vi "createSheet.vi"(6 "Set as active (T)":bool=TRUE, 8 "error in (no error)":errorcluster, 10 "SheetName":string, 11 "MS-Excel in":refnum<class "MS-Excel.lvclass">) -> (0 "error out":errorcluster, 1 "Created?":bool, 2 "Created Sheet Name":string, 3 "MS-Excel out":refnum<class "MS-Excel.lvclass">)   [LabVIEW 2020, in "LabVIEW NPOI.lvlib" / "MS-Excel.lvclass"]
uses:
  MS-Excel.lvclass
  D:/Benjamin/Documents/Perso/Code/WC/LabVIEW_NPOI/lib/NPOI 2.1.1/NPOI.dll
  lib/NPOI 2.1.1/NPOI.dll
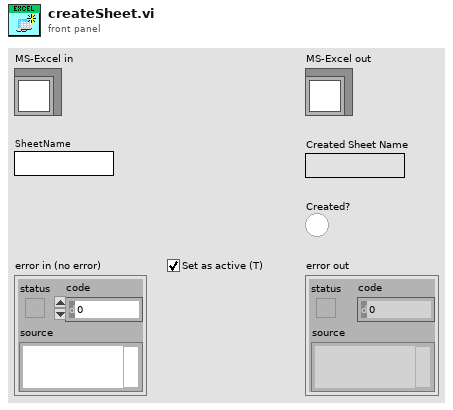
[diagram p1: front panel]
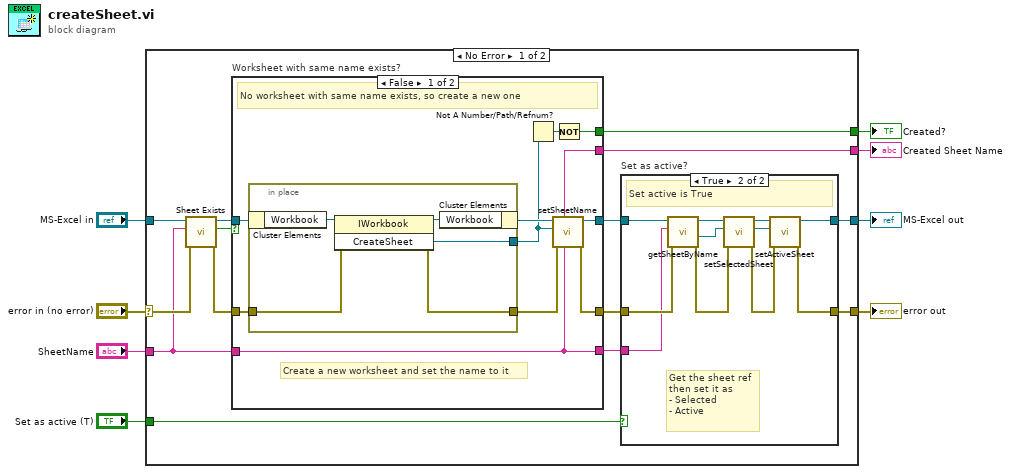
[diagram p0: block diagram]
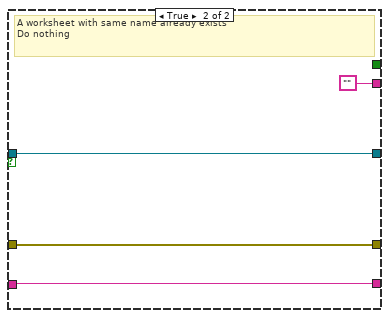
[diagram p3: hidden frame]
diagram:
  n1 = case shown="No Error" "error in (no error)" {
    selector: "error in (no error)" -> [w19 w55]
    tunnel: [w13 w55] -> w7
    tunnel: [w12 w54] -> w5
    tunnel: "MS-Excel in" -> [w22 w54]
    tunnel: "SheetName" -> [w17 _]
    tunnel: "Set as active (T)" -> [w11 _]
    tunnel: [w21 _] -> w2
    tunnel: [w9 _] -> w1
    frame No Error {
      n2 = call "Sheet Exists.vi"("error in (no error)"=w19, "Sheet Name"=w17, "MS-Excel in"=w22) -> ("error out"=w18:errorcluster, "Exists"=w16:bool, "MS-Excel out"=w20:refnum<class "MS-Excel.lvclass">)  [unwired: 6 in]
      n3 = case "Worksheet with same name exists?" shown="False" w16 {
        tunnel: [w36 w53] -> w15
        tunnel: [w37 w52] -> w14
        tunnel: [w42 _] -> w21
        tunnel: w20 -> [w39 w53]
        tunnel: w17 -> [w35 w51]
        tunnel: w18 -> [w38 w52]
        tunnel: [w35 w51] -> w10
        tunnel: [w35 "" ("SheetName")] -> w9
        frame False {
          # "Create a new worksheet and set the name to it"
          # "No worksheet with same name exists, so create a new one"
          n4 = in-place {
            in-place-border: w38 -> [w48]
            in-place-border: [w46] -> w40
            in-place-border: [w45] -> w41
            n5 = in-place-cluster #1(w39) -> ("Workbook"=w49:refnum<k24>)
            n6 = invoke class="IWorkbook" method="CreateSheet"(reference=w49, error in=w48) -> (reference out=w47:refnum<k24>, error out=w46:errorcluster, "CreateSheet"=w45:refnum<k24>)  [unwired: 1 in]
            n7 = in-place-cluster #1("Workbook"=w47) -> (w44:refnum<class "MS-Excel.lvclass">)
          }
          n8 = Not A Number/Path/Refnum?(number/path/refnum=w41) -> (NaN/Path/Refnum?=w43:bool)
          n9 = call-dynamic "setSheetName.vi"("Sheet Name"=w35, "error in (no error)"=w40, "SheetRef"=w41, "MS-Excel in"=w44) -> ("error out"=w37:errorcluster, "MS-Excel out"=w36:refnum<class "MS-Excel.lvclass">)  [unwired: 6 in]
          n10 = Not(x=w43) -> (.not. x?=w42:bool)
        }
        frame True {
          # "A worksheet with same name already exists\nDo nothing"
        }
      }
      n11 = case "Set as active?" shown="True" w11 {
        tunnel: w15 -> [w24 w30]
        tunnel: w14 -> [w23 w28]
        tunnel: [w24 w33] -> w12
        tunnel: [w23 w31] -> w13
        tunnel: w10 -> [_ w25]
        frame False {
          # "Set active is False"
        }
        frame True {
          # "Get the sheet ref \nthen set it as \n- Selected\n- Active"
          # "Set active is True"
          n12 = call-dynamic "getSheetByName.vi"("error in (no error)"=w28, "Sheet Name"=w25, "MS-Excel in"=w30) -> ("error out"=w27:errorcluster, "Sheet Ref"=w26:refnum<k24>, "MS-Excel out"=w29:refnum<class "MS-Excel.lvclass">)  [unwired: 5 in, 1 out]
          n13 = call-dynamic "setSelectedSheet.vi"("error in (no error)"=w27, "Sheet Ref"=w26, "MS-Excel in"=w29) -> ("error out"=w32:errorcluster, "MS-Excel out"=w34:refnum<class "MS-Excel.lvclass">)  [unwired: 7 in]
          n14 = call-dynamic "setActiveSheet.vi"("error in (no error)"=w32, "Sheet Ref"=w26, "MS-Excel in"=w34) -> ("error out"=w31:errorcluster, "MS-Excel out"=w33:refnum<class "MS-Excel.lvclass">)  [unwired: 7 in]
        }
      }
    }
    frame Error {
    }
  }
  "error out" <- w7
  "MS-Excel out" <- w5
  "Created?" <- w2
  "Created Sheet Name" <- w1
